vi "Set Slave Node-ID.vi"(8 "error in":errorcluster, 10 "Slave Node-ID":u8 format="%.0x", 11 "Interactor in":refnum<class "Interactor.lvclass">) -> (0 "error out":errorcluster, 3 "Interactor out":refnum<class "Interactor.lvclass">)   [LabVIEW 2024, in "Interactor.lvlib" / "Interactor.lvclass"]
uses:
  Interactor.lvclass
  Interactor.lvclass/Interactor.ctl
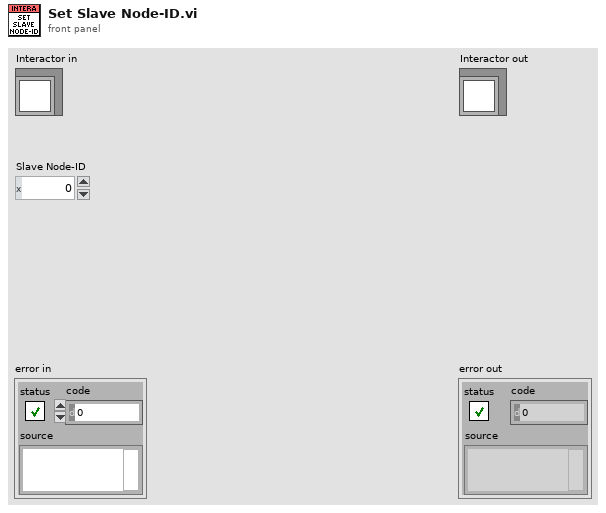
[diagram p1: front panel]
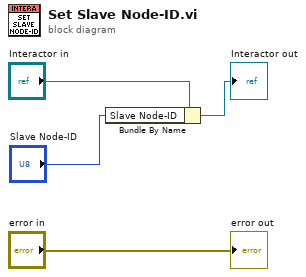
[diagram p0: block diagram]
diagram:
  n1 = Bundle By Name(cluster="Interactor in", "Slave Node-ID"="Slave Node-ID") -> (→"Interactor out":refnum<class "Interactor.lvclass">)
  "error out" <- "error in"
